vi "Forward Pass (LSTM).vi"() -> ()   [LabVIEW 2014]
uses:
  <vilib>/Analysis/NI_AALBase.lvlib
  <vilib>/Analysis/baseanly.llb/Real A x B.vi
  <vilib>/Analysis/Matrix/NI_Matrix.lvlib
  <vilib>/Analysis/Matrix/Numeric/Add/Add - RM,RM.vi
  <vilib>/Analysis/Matrix/Datatypes/RealMatrix.ctl
panel:
  out "Wco * c[t]":T1
  out "Wxo * x[t]":T1=[[2.5697], [-0.172737]]
  out "Who * h[t-1]":T1
  out "Wxc * x[t]":T1=[[2.5697], [-0.172737]]
  out "Whc * h[t-1]":T1
  out "Wcf * c[t-1]":T1
  out "Wxf * x[t]":T1=[[2.5697], [-0.172737]]
  out "Whf * h[t-1]":T1
  out "Wci * c[t-1]":T1
  out "h[t]":T1=[[0.9959896974183432], [-0.973683146441647]]
  out "tanh(c[t])":T1
  out "Wco * c[t]":T1
  out "Wxo * x[t] + Who * h[t-1]\n + Wco * c[t] + bo":T1=[[0.5353143], [-1.98598657]]
  out "o[t]":T1=[[0.9959896974183432], [-0.973683146441647]]
  out "Wxo* x[t]":T1=[[2.5697], [-0.172737]]
  out "Who * h[t-1]":T1
  out "c[t]":T1
  out "f[t] * c[t-1]":T1=[[2.5697], [-0.172737]]
  out "i[t] * h_hat[t]":T1
  out "c_hat[t]":T1=[[0.9959896974183432], [-0.973683146441647]]
  out "Wxc * x[t] + Whc * h[t-1] + bc":T1=[[0.5353143], [-1.98598657]]
  out "Wxc * x[t]":T1=[[2.5697], [-0.172737]]
  out "Whc * h[t-1]":T1
  out "Wcf * c[t-1]":T1
  out "Whx * x[t] + Whf * h[t-1]\n + Wcf * c[t-1] + bf":T1=[[0.5353143], [-1.98598657]]
  out "f[t]":T1=[[0.9959896974183432], [-0.973683146441647]]
  out "Wxf * x[t]":T1=[[2.5697], [-0.172737]]
  out "Whf * h[t-1]":T1
  in  "c[t-1]":T1=[[0.0], [0.0]]
  out "Wci * c[t-1]":T1
  out "Whx * x[t] + Whi * h[t-1]\n + Wci * c[t-1] + bi":T1=[[0.5353143], [-1.98598657]]
  out "p[t]":T1=[[0.20283716485987413], [0.10368793196933078], [0.6934749031707951]]
  out "i[t]":T1=[[0.9959896974183432], [-0.973683146441647]]
  in  "x[t]":T1=[[0.0], [1.0], [0.0]]
  in  "h[t-1]":T1=[[0.0], [0.0]]
  in  "LSTM params":T2={"Wxi"=[[0.57813, 2.5697, -0.0219857], [-2.4696, -0.172737, 2.44961362]], "Whi"=[[-1.39960002, 0.96174453], [0.36456552, -0.47706397]], "Wci"=[[-0.6486, 0.76469], [-1.77899, 0.38803572], [-0.1309121, -0.333988]], "bi"=[[0.5353143], [-1.98598657]], "Wxf"=[[0.57813, 2.5697, -0.0219857], [-2.4696, -0.172737, 2.44961362]], "Whf"=[[-0.6486, 0.76469], [-1.77899, 0.38803572], [-0.1309121, -0.333988]], "Wcf"=[[-1.39960002, 0.96174453], [0.36456552, -0.47706397]], "bf"=[[0.5353143], [-1.98598657]], "Wxc"=[[0.57813, 2.5697, -0.0219857], [-2.4696, -0.172737, 2.44961362]], "Whc"=[[-0.6486, 0.76469], [-1.77899, 0.38803572], [-0.1309121, -0.333988]], "bc"=[[0.5353143], [-1.98598657]], "Wxo"=[[0.57813, 2.5697, -0.0219857], [-2.4696, -0.172737, 2.44961362]], "Who"=[[-0.6486, 0.76469], [-1.77899, 0.38803572], [-0.1309121, -0.333988]], "Wco"=[[-1.39960002, 0.96174453], [0.36456552, -0.47706397]], "bo"=[[-0.52841737], [-0.44032028], [-0.8844819]]}
  out "Why * h[t]":T1=[[-1.3905646829980003], [-2.1496795525916084], [0.1948113838463529]]
  out "Wxi * x[t]":T1=[[2.5697], [-0.172737]]
  out "y[t] = Why * h[t] + by":T1=[[-1.9189820529980004], [-2.5899998325916083], [-0.6896705161536472]]
  out "sum":dbl=0.7235176863832331
  out "e^y[t]":T1=[[0.14675627623195056], [0.07502005264431227], [0.5017413575069702]]
  out "Whi * h[t-1]":T1
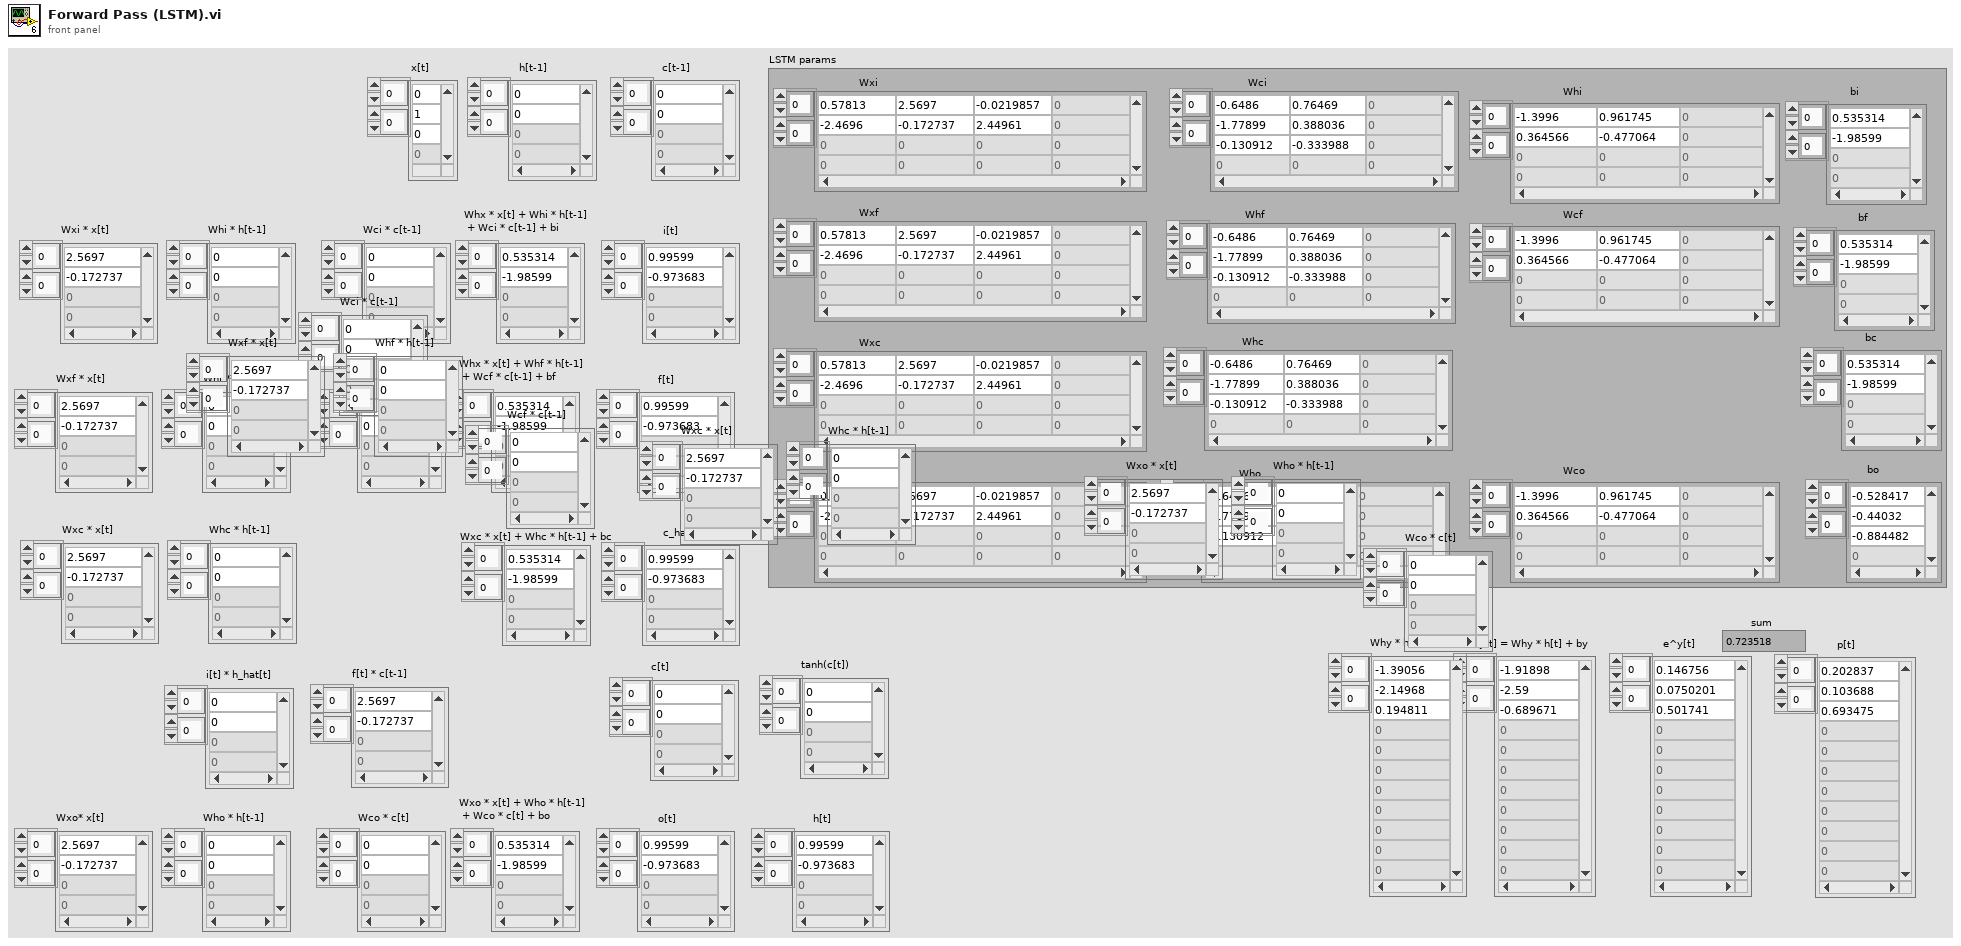
[diagram p1: front panel]
types:
  T1 = typedef "NI_Matrix.lvlib/RealMatrix.ctl" = dbl[][]
  T2 = cluster{"Wxi":T1, "Whi":T1, "Wci":T1, "bi":T1, "Wxf":T1, "Whf":T1, "Wcf":T1, "bf":T1, "Wxc":T1, "Whc":T1, "bc":T1, "Wxo":T1, "Who":T1, "Wco":T1, "bo":T1}
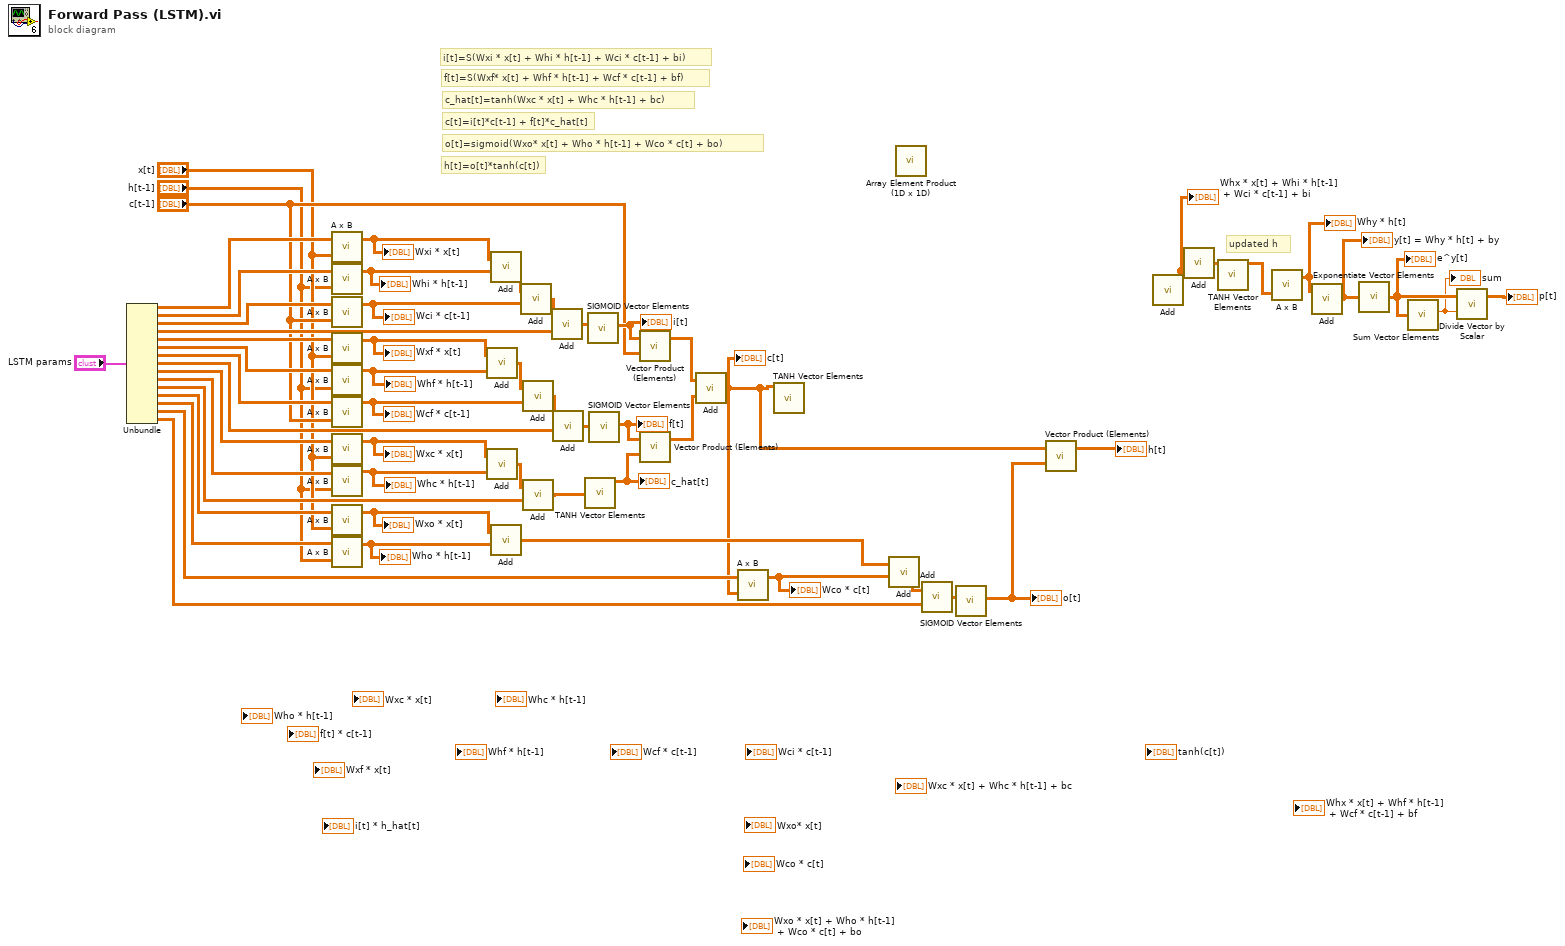
[diagram p0: block diagram]
diagram:
  # "h[t]=o[t]*tanh(c[t])"
  # "o[t]=sigmoid(Wxo* x[t] + Who * h[t-1] + Wco * c[t] + bo)"
  # "c_hat[t]=tanh(Wxc * x[t] + Whc * h[t-1] + bc)"
  # "c[t]=i[t]*c[t-1] + f[t]*c_hat[t]"
  # "f[t]=S(Wxf* x[t] + Whf * h[t-1] + Wcf * c[t-1] + bf)"
  # "i[t]=S(Wxi * x[t] + Whi * h[t-1] + Wci * c[t-1] + bi)"
  # "updated h"
  n1 = Unbundle("LSTM params") -> ("Wxi"=w56:T1, "Whi"=w57:T1, "Wci"=w46:T1, "bi"=w35:T1, "Wxf"=w34:T1, "Whf"=w33:T1, "Wcf"=w32:T1, "bf"=w31:T1, "Wxc"=w25:T1, "Whc"=w24:T1, "bc"=w23:T1, "Wxo"=w9:T1, "Who"=w8:T1, "Wco"=w7:T1, "bo"=w6:T1)
  n2 = call-poly <vilib>:"A x B.vi"("B"="x[t]", "A"=w56) -> ("A x B"=w45:T1)  [unwired: 1 out]
  "Wxi * x[t]" <- w45
  n3 = call-poly <vilib>:"A x B.vi"("B"="h[t-1]", "A"=w57) -> ("A x B"=w44:T1)  [unwired: 1 out]
  "Whi * h[t-1]" <- w44
  n4 = call-poly <vilib>:"A x B.vi"("B"="c[t-1]", "A"=w46) -> ("A x B"=w42:T1)  [unwired: 1 out]
  "Wci * c[t-1]" <- w42
  n5 = call-poly <vilib>:"A x B.vi"("B"="x[t]", "A"=w34) -> ("A x B"=w40:T1)  [unwired: 1 out]
  "Wxf * x[t]" <- w40
  n6 = call-poly <vilib>:"A x B.vi"("B"="h[t-1]", "A"=w33) -> ("A x B"=w39:T1)  [unwired: 1 out]
  "Whf * h[t-1]" <- w39
  n7 = call-poly <vilib>:"A x B.vi"("B"="c[t-1]", "A"=w32) -> ("A x B"=w37:T1)  [unwired: 1 out]
  "Wcf * c[t-1]" <- w37
  n8 = call-poly <vilib>:"A x B.vi"("B"="x[t]", "A"=w25) -> ("A x B"=w28:T1)  [unwired: 1 out]
  "Wxc * x[t]" <- w28
  n9 = call-poly <vilib>:"A x B.vi"("B"="h[t-1]", "A"=w24) -> ("A x B"=w27:T1)  [unwired: 1 out]
  "Whc * h[t-1]" <- w27
  n10 = call-poly <vilib>:"A x B.vi"("B"="x[t]", "A"=w9) -> ("A x B"=w15:T1)  [unwired: 1 out]
  "Wxo * x[t]" <- w15
  n11 = call-poly <vilib>:"A x B.vi"("B"="h[t-1]", "A"=w8) -> ("A x B"=w14:T1)  [unwired: 1 out]
  "Who * h[t-1]" <- w14
  n12 = call-poly <vilib>:"Add.vi"("Real Matrix B"=w39, "Real Matrix A"=w40) -> ("A + B"=w38:T1)
  n13 = call-poly <vilib>:"Add.vi"("Real Matrix B"=w27, "Real Matrix A"=w28) -> ("A + B"=w26:T1)
  n14 = call-poly <vilib>:"Add.vi"("Real Matrix B"=w44, "Real Matrix A"=w45) -> ("A + B"=w43:T1)
  n15 = call-poly <vilib>:"Add.vi"("Real Matrix B"=w14, "Real Matrix A"=w15) -> ("A + B"=w13:T1)
  n16 = call-poly <vilib>:"Add.vi"("Real Matrix B"=w42, "Real Matrix A"=w43) -> ("A + B"=w41:T1)
  n17 = call-poly <vilib>:"Add.vi"("Real Matrix B"=w37, "Real Matrix A"=w38) -> ("A + B"=w36:T1)
  n18 = call-poly <vilib>:"Add.vi"("Real Matrix B"=w23, "Real Matrix A"=w26) -> ("A + B"=w22:T1)
  n19 = call-poly <vilib>:"Add.vi"("Real Matrix B"=w35, "Real Matrix A"=w41) -> ("A + B"=w30:T1)
  n20 = call-poly <vilib>:"Add.vi"("Real Matrix B"=w31, "Real Matrix A"=w36) -> ("A + B"=w29:T1)
  n21 = call "TANH Vector Elements.vi"("X"=w22) -> ("tanh(X)"=w18:T1)  [unwired: 10 in]
  "c_hat[t]" <- w18
  n22 = call "SIGMOID Vector Elements.vi"("X"=w30) -> ("sigmoid(X)"=w21:T1)  [unwired: 18 in]
  "i[t]" <- w21
  n23 = call "SIGMOID Vector Elements.vi"("X"=w29) -> ("sigmoid(X)"=w19:T1)  [unwired: 18 in]
  "f[t]" <- w19
  n24 = call "Vector Product (Elements).vi"("X"=w21, "Y"="c[t-1]") -> ("X*Y"=w17:T1)  [unwired: 17 in]
  n25 = call "Vector Product (Elements).vi"("X"=w19, "Y"=w18) -> ("X*Y"=w16:T1)  [unwired: 17 in]
  n26 = call-poly <vilib>:"Add.vi"("Real Matrix B"=w16, "Real Matrix A"=w17) -> ("A + B"=w3:T1)
  "c[t]" <- w3
  n27 = call-poly <vilib>:"A x B.vi"("B"=w3, "A"=w7) -> ("A x B"=w12:T1)  [unwired: 1 out]
  "Wco * c[t]" <- w12
  n28 = call "TANH Vector Elements.vi"("X"=w3) -> ()  [unwired: 10 in, 1 out]
  n29 = call-poly <vilib>:"Add.vi"("Real Matrix B"=w12, "Real Matrix A"=w13) -> ("A + B"=w11:T1)
  n30 = call "Array Element Product (1D x 1D).vi"() -> ()  [unwired: 19 in, 1 out]
  n31 = call-poly <vilib>:"Add.vi"("Real Matrix B"=w6, "Real Matrix A"=w11) -> ("A + B"=w10:T1)
  n32 = call "SIGMOID Vector Elements.vi"("X"=w10) -> ("sigmoid(X)"=w2:T1)  [unwired: 18 in]
  "o[t]" <- w2
  n33 = call "Vector Product (Elements).vi"("X"=w3, "Y"=w2) -> ("X*Y"=→"h[t]":T1)  [unwired: 17 in]
  n34 = call-poly <vilib>:"Add.vi"() -> ("A + B"=w47:T1)  [unwired: 2 in]
  "Whx * x[t] + Whi * h[t-1]\n + Wci * c[t-1] + bi" <- w47
  n35 = call-poly <vilib>:"Add.vi"("Real Matrix B"=w47) -> ("A + B"=w52:T1)  [unwired: 1 in]
  n36 = call "TANH Vector Elements.vi"("X"=w52) -> ("tanh(X)"=w53:T1)  [unwired: 10 in]
  n37 = call-poly <vilib>:"A x B.vi"("B"=w53) -> ("A x B"=w51:T1)  [unwired: 1 in, 1 out]
  "Why * h[t]" <- w51
  n38 = call-poly <vilib>:"Add.vi"("Real Matrix A"=w51) -> ("A + B"=w54:T1)  [unwired: 1 in]
  "y[t] = Why * h[t] + by" <- w54
  n39 = call "Exponentiate Vector Elements.vi"("X"=w54) -> ("exp(X)"=w50:T1)
  "e^y[t]" <- w50
  n40 = call "Sum Vector Elements.vi"("A x B"=w50) -> ("Numeric"=w49:dbl)
  "sum" <- w49
  n41 = call "Divide Vector by Scalar.vi"("Vector"=w50, "x"=w49) -> ("Scaled Vector"=→"p[t]":T1)  [unwired: 17 in]
